vi "Ethernet Reader Modified.vi"() -> ()   [LabVIEW 2020]
doc: "This example creates a frame input stream session, reads frames at a set interval, and displays all the received frames from the latest read on the front panel."
uses:
  <resource>/objmgr/xnet.rc
  <vilib>/userdefined/xnetEnetEptRxFilterElement.ctl
  <vilib>/xnet/xnet.llb/XNET Create Session (Frame Input Stream).vi
  JLR/emea-tra-JLR-Synchronization-PoC/PoC_LV2020/States.ctl
  <vilib>/xnet/xnet.llb/XNET Read (State Time Current).vi
  JLR/emea-tra-JLR-Synchronization-PoC/PoC_LV2020/Data.ctl
  <vilib>/xnet/xnet.llb/XNET Read (Frame Ethernet).vi
  <vilib>/xnet/xnet.llb/XNET Read (State Time Trigger).vi
  <instrlib>/niSync/niSync.llb/niSync Set Time (Manual).vi
  <instrlib>/niSync/niSync.llb/niSync Initialize (Default).vi
  <vilib>/xnet/xnet.llb/XNET Frame Type Ethernet.ctl
  <vilib>/xnet/xnet.llb/XNET Frame Ethernet.ctl
panel:
  out "error out":errorcluster
  out "local time current":timestamp
  out "NI Sync Time":timestamp
  in  "Can Interface":refnum<k21>="LIN1"
  in  "Generate Trigger":bool
  out "Port State":u32(ring)=3 items=["Disabled"=3, "Master"=6, "Passive"=7, "Slave"=9]
  out "Synced?":bool
  out "Offset From Master (ns) 2":i64
  out "Frame Data (as hex string) Array 2":string[](array[string])
  out "Ethernet Read Frame Array 2":T1[](array[typedef]) {"fcs" format="%08x"; "network timestamp" format="%<%.7X\n%x>T"; "frame data" format="%x"; "local timestamp" format="%<%.7X\n%x>T"; "type" items=["Ethernet Data"=0, "Delay"=225, "Future Time Wait"=226]}
  out "Array Size 2":i32
  out "Number of Frames Received":u64
  in  "NI Sync Name":tag="Dev1"
  in  "Interface":refnum<k21>="ENET1"
  out "Time Diff (Sync vs Xnet) (s)":dbl format="%#.6f"
  in  "Stop 2":bool
  out "?":T3 {"Time Trigger Received" format="%<%.6X\n%x>T"}
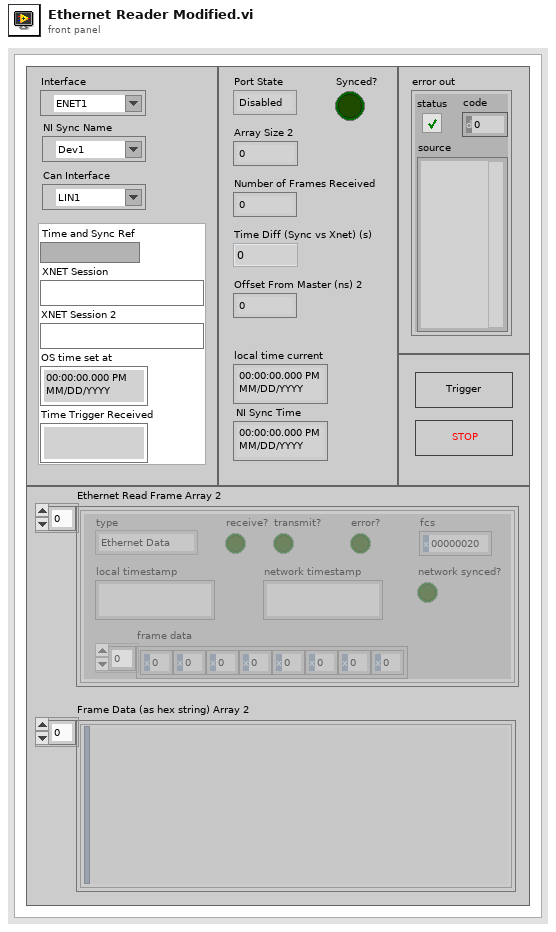
[diagram p1: front panel]
types:
  T1 = typedef "XNET Frame Ethernet.ctl" = cluster{"local timestamp":timestamp, "network timestamp":timestamp, "frame data":u8[], "fcs":u32, "type":T2, "network synced?":bool, "receive?":bool, "transmit?":bool, "error?":bool}
  T2 = typedef "XNET Frame Type Ethernet.ctl" = u16
  T3 = typedef "Data.ctl" = cluster{"Time and Sync Ref":refnum<k15>, "XNET Session":refnum<k21>, "XNET Session 2":refnum<k21>, "OS time set at":timestamp, "Time Trigger Received":timestamp}
  T4 = typedef "States.ctl" = enum16{"Init 8523", "Init 6683", "Sync 8523", "PPS+Trigger", "Set Sync Time", "Init 8510", "Adjust XNET time", "Idle", "Error"}
  T5 = typedef "xnetEnetEptRxFilterElement.ctl" = cluster{"use VID?":bool, "VID":u16, "use priority?":bool, "priority":u8, "use destination MAC?":bool, "destination MAC":string}
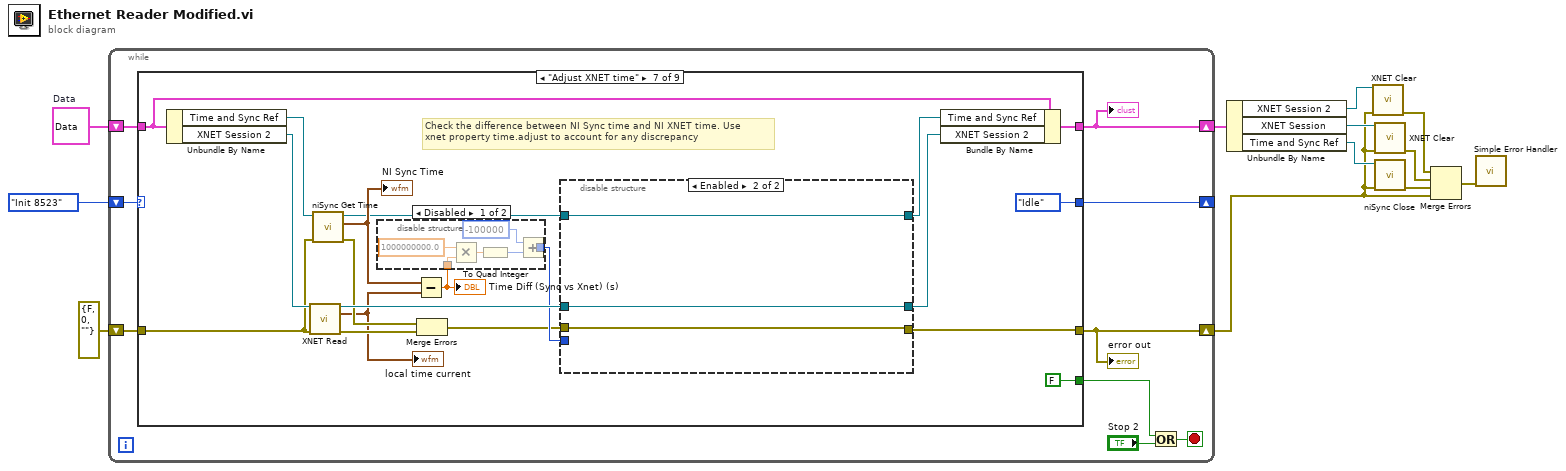
[diagram p0: block diagram]
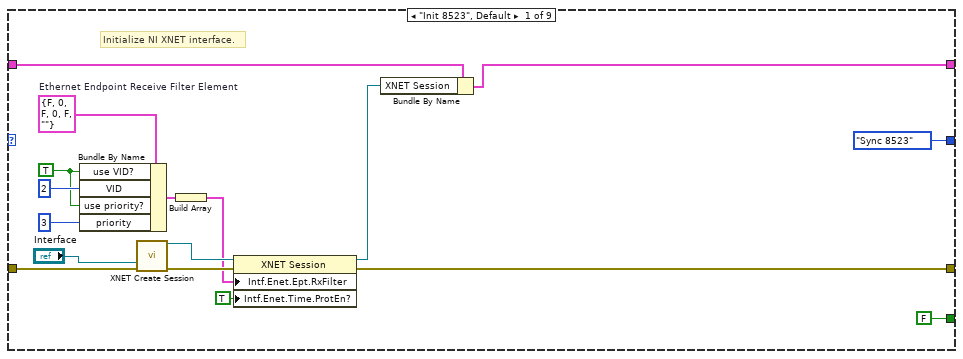
[diagram p2: hidden frame]
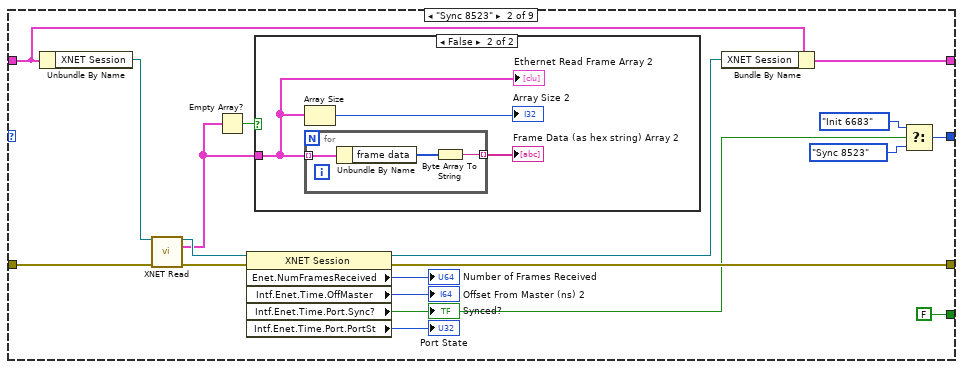
[diagram p3: hidden frame]
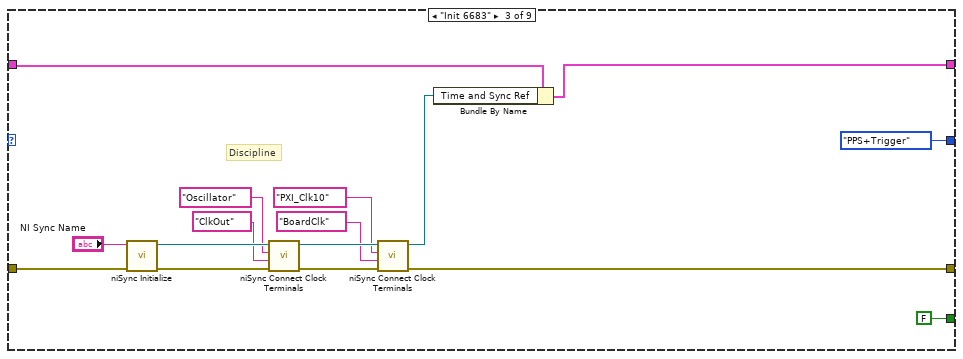
[diagram p5: hidden frame]
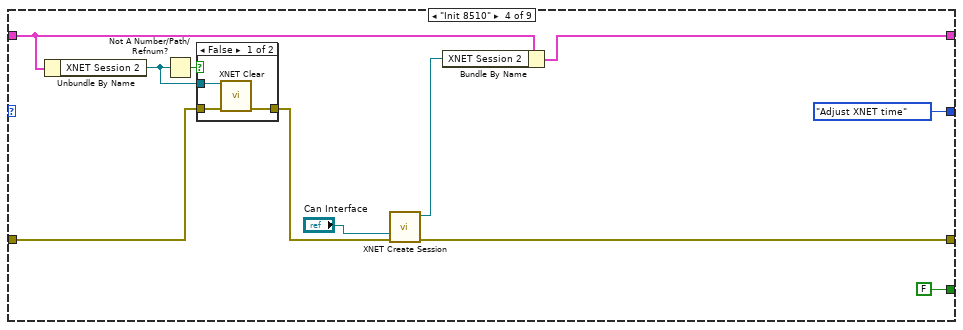
[diagram p6: hidden frame]
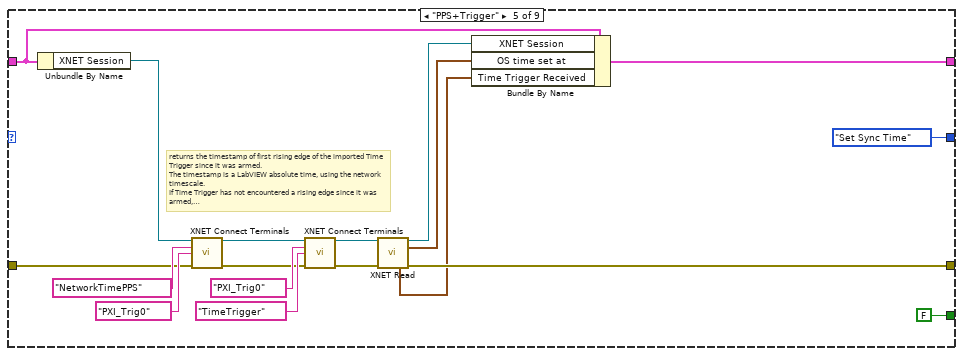
[diagram p8: hidden frame]
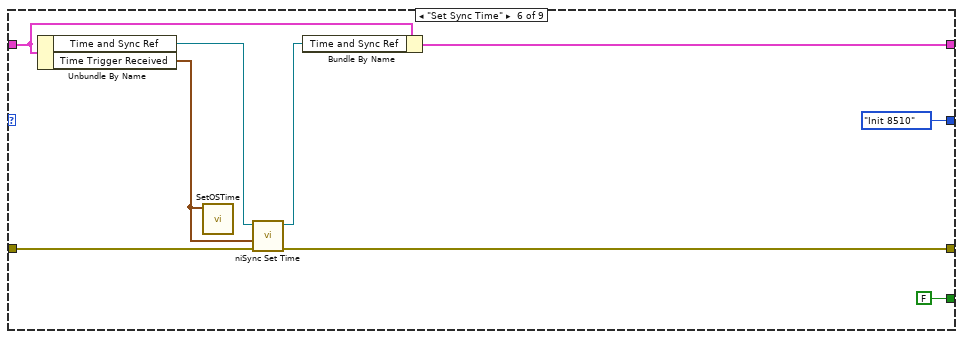
[diagram p9: hidden frame]
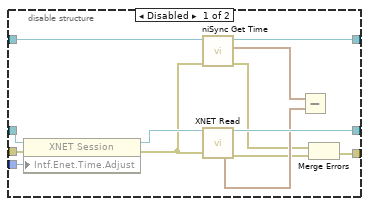
[diagram p11: hidden frame]
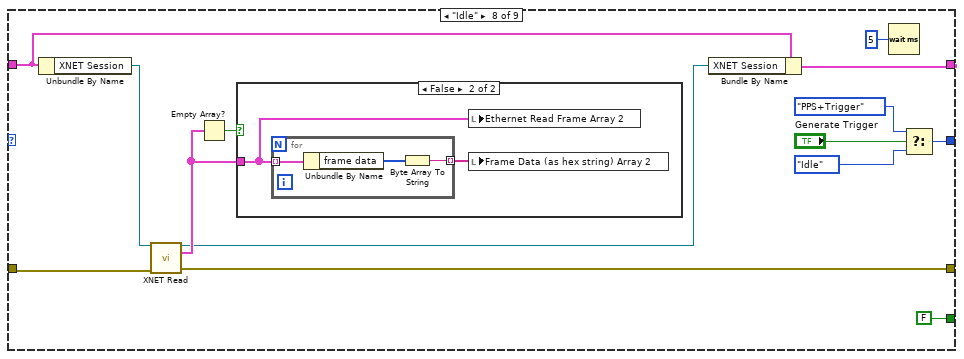
[diagram p12: hidden frame]
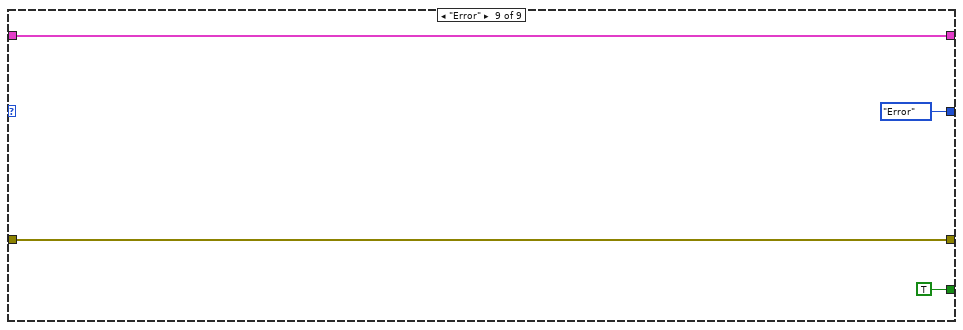
[diagram p14: hidden frame]
diagram:
  w6 = T3 {"Time and Sync Ref"="", "XNET Session"="", "XNET Session 2"="", "OS time set at"=timestamp(0 s since 1904-01-01), "Time Trigger Received"=timestamp(0 s since 1904-01-01)}  # Data
  n1 = while {
    shift-right: [w18] -> _
    shift-left: States."Init 8523" -> [w21]
    shift-right: [w13] -> w3
    shift-left: errorcluster {"status"=FALSE, "code"=0, "source"=""} ("error out") -> [w19]
    shift-right: [w15] -> w9
    shift-left: w6 -> [w20]
    stop <- w17 stop-if-true
    n2 = case shown="\"Adjust XNET time\"" w21 {
      tunnel: w20 -> [w38 w46 w69 w83 w101 w116 w124 w167 w181]
      tunnel: [w25 w52 w65 w86 w97 w115 w126 w165 w183] -> w13
      tunnel: w19 -> [w26 w43 w68 w80 w98 w118 w132 w166 w183]
      tunnel: [w36 w47 w67 w84 w100 w117 w133 w168 w181] -> w15
      tunnel: [States."Sync 8523" w49 States."PPS+Trigger" States."Adjust XNET time" States."Set Sync Time" States."Init 8510" States."Idle" w173 States."Error"] -> w18
      tunnel: [FALSE ("Intf.Enet.Time.Port.Sync?") FALSE ("Intf.Enet.Time.Port.Sync?") FALSE ("Intf.Enet.Time.Port.Sync?") FALSE ("Intf.Enet.Time.Port.Sync?") FALSE ("Intf.Enet.Time.Port.Sync?") FALSE ("Intf.Enet.Time.Port.Sync?") FALSE ("Intf.Enet.Time.Port.Sync?") FALSE ("Intf.Enet.Time.Port.Sync?") TRUE ("Intf.Enet.Time.Port.Sync?")] -> w14
      frame "Init 8523", Default {
        w28 = TRUE ("use VID?")
        w29 = T5 {"use VID?"=FALSE, "VID"=0, "use priority?"=FALSE, "priority"=0, "use destination MAC?"=FALSE, "destination MAC"=""}  # Ethernet Endpoint Receive Filter Element
        # "Initialize NI XNET interface."
        n3 = Bundle By Name(cluster=w29, "use VID?"=w28, "VID"=u16 2 ("VID 2"), "use priority?"=w28, "priority"=u8 3 ("priority 2")) -> (w32:T5)
        n4 = call-poly <vilib>:"XNET Create Session.vi"("interface"="Interface", "error in (no error)"=w26) -> ("session out"=w34:refnum<k21>, "error out"=w35:errorcluster)  [unwired: 12 in]
        n5 = Build Array(w32) -> (w33:T5[])
        n6 = property class="XNET Session"(reference=w34, error in=w35, "Intf.Enet.Ept.RxFilter"=w33, "Intf.Enet.Time.ProtEn?"=TRUE ("Interface:Ethernet:Time Sync:Protocol Enabled?")) -> (reference out=w24:refnum<k21>, error out=w25:errorcluster)
        n7 = Bundle By Name(cluster=w38, "XNET Session"=w24) -> (w36:T3)
      }
      frame "Sync 8523" {
        n8 = Unbundle By Name(w46) -> ("XNET Session"=w45:refnum<k21>)
        n9 = call-poly <vilib>:"XNET Read.vi"("session in"=w45, "error in (no error)"=w43) -> ("session out"=w42:refnum<k21>, "data"=w41:T1[], "error out"=w44:errorcluster)  [unwired: 10 in, 1 out]
        n10 = Empty Array?(array=w41) -> (empty?=w55:bool)
        n11 = property class="XNET Session"(reference=w42, error in=w44) -> (reference out=w48:refnum<k21>, error out=w52:errorcluster, "Enet.NumFramesReceived"=→"Number of Frames Received":u64, "Intf.Enet.Time.OffMaster"=→"Offset From Master (ns) 2":i64, "Intf.Enet.Time.Port.Sync?"=w40:bool, "Intf.Enet.Time.Port.PortSt"=→"Port State":u32)
        "Synced?" <- w40
        n12 = case shown="False" w55 {
          tunnel: w41 -> [_ w57]
          frame True {
          }
          frame False {
            n13 = Array Size(array=w57) -> (size(s)=→"Array Size 2":i32)
            n14 = for {
              tunnel: [w62] -> w59 mode=indexing
              tunnel: w57 -> [w61] mode=indexing
              n15 = Unbundle By Name(w61) -> ("frame data"=w60:u8[])
              n16 = Byte Array To String(unsigned byte array=w60) -> (string=w62:string)
            }
            "Frame Data (as hex string) Array 2" <- w59
            "Ethernet Read Frame Array 2" <- w57
          }
        }
        n17 = Bundle By Name(cluster=w46, "XNET Session"=w48) -> (w47:T3)
        n18 = Select(t=States."Init 6683", s=w40, f=States."Sync 8523") -> (s? t:f=w49:T4)
      }
      frame "Init 6683" {
        # "Discipline"
        n19 = call-poly <instrlib>:"niSync Initialize.vi"("error in (no error)"=w68, "resource name"="NI Sync Name") -> ("error out"=w78:errorcluster, "instrument handle out"=w77:refnum<k15>)  [unwired: 8 in]
        n20 = call <instrlib>:"niSync Connect Clock Terminals.vi"("error in (no error)"=w78, "destination terminal"="ClkOut", "source terminal"="Oscillator", "instrument handle"=w77) -> ("error out"=w75:errorcluster, "instrument handle out"=w76:refnum<k15>)  [unwired: 6 in]
        n21 = call <instrlib>:"niSync Connect Clock Terminals.vi"("error in (no error)"=w75, "destination terminal"="BoardClk", "source terminal"="PXI_Clk10", "instrument handle"=w76) -> ("error out"=w65:errorcluster, "instrument handle out"=w64:refnum<k15>)  [unwired: 6 in]
        n22 = Bundle By Name(cluster=w69, "Time and Sync Ref"=w64) -> (w67:T3)
      }
      frame "Init 8510" {
        n23 = Unbundle By Name(w83) -> ("XNET Session 2"=w81:refnum<k21>)
        n24 = Not A Number/Path/Refnum?(number/path/refnum=w81) -> (NaN/Path/Refnum?=w82:bool)
        n25 = case shown="False" w82 {
          tunnel: w81 -> [w92 _]
          tunnel: w80 -> [w91 w93]
          tunnel: [w90 w93] -> w79
          frame False {
            n26 = call <vilib>:"XNET Clear.vi"("session in"=w92, "error in (no error)"=w91) -> ("error out"=w90:errorcluster)  [unwired: 13 in]
          }
          frame True {
          }
        }
        n27 = call-poly <vilib>:"XNET Create Session.vi"("interface"="Can Interface", "error in (no error)"=w79) -> ("session out"=w85:refnum<k21>, "error out"=w86:errorcluster)  [unwired: 1 in, 11 out]
        n28 = Bundle By Name(cluster=w83, "XNET Session 2"=w85) -> (w84:T3)
      }
      frame "PPS+Trigger" {
        # "returns the timestamp of first rising edge of the imported Time Trigger since it was armed. \nThe timestamp is a LabVIEW absolute time, using the network timescale. \nIf Time Trigger has not encountered a rising edge since it was armed, \nnetwork time trigger returns zero (an invalid timestamp)."
        n29 = Unbundle By Name(w101) -> ("XNET Session"=w103:refnum<k21>)
        n30 = call <vilib>:"XNET Connect Terminals.vi"("session in"=w103, "source terminal"=tag "NetworkTimePPS", "destination terminal"=tag "PXI_Trig0", "error in (no error)"=w98) -> ("session out"=w106:refnum<k21>, "error out"=w107:errorcluster)  [unwired: 10 in]
        n31 = call <vilib>:"XNET Connect Terminals.vi"("session in"=w106, "source terminal"=tag "PXI_Trig0", "destination terminal"=tag "TimeTrigger", "error in (no error)"=w107) -> ("session out"=w102:refnum<k21>, "error out"=w104:errorcluster)  [unwired: 10 in]
        n32 = call-poly <vilib>:"XNET Read.vi"("session in"=w102, "error in (no error)"=w104) -> ("session out"=w111:refnum<k21>, "local time trigger"=w95:timestamp, "network time trigger"=w94:timestamp, "error out"=w97:errorcluster)  [unwired: 9 in, 1 out]
        n33 = Bundle By Name(cluster=w101, "XNET Session"=w111, "OS time set at"=w95, "Time Trigger Received"=w94) -> (w100:T3)
      }
      frame "Set Sync Time" {
        n34 = Unbundle By Name(w116) -> ("Time and Sync Ref"=w119:refnum<k15>, "Time Trigger Received"=w112:timestamp)
        n35 = call "SetOSTime.vi"("OS time"=w112) -> ()  [unwired: 10 in, 1 out]
        n36 = call-poly <instrlib>:"niSync Set Time.vi"("error in (no error)"=w118, "initial time"=w112, "instrument handle"=w119) -> ("error out"=w115:errorcluster, "instrument handle out"=w114:refnum<k15>)  [unwired: 7 in]
        n37 = Bundle By Name(cluster=w116, "Time and Sync Ref"=w114) -> (w117:T3)
      }
      frame "Adjust XNET time" {
        # "Check the difference between NI Sync time and NI XNET time. Use\nxnet property time.adjust to account for any discrepancy"
        n38 = Unbundle By Name(w124) -> ("Time and Sync Ref"=w134:refnum<k15>, "XNET Session 2"=w135:refnum<k21>)
        n39 = call-poly <vilib>:"XNET Read.vi"("session in"=w135, "error in (no error)"=w132) -> ("session out"=w137:refnum<k21>, "local time current"=w123:timestamp, "error out"=w136:errorcluster)  [unwired: 9 in, 2 out]
        "local time current" <- w123
        n40 = call <instrlib>:"niSync Get Time.vi"("error in (no error)"=w132, "instrument handle"=w134) -> ("error out"=w131:errorcluster, "time"=w139:timestamp, "instrument handle out"=w128:refnum<k15>)  [unwired: 5 in]
        "NI Sync Time" <- w139
        n41 = Subtract(x=w139, y=w123) -> (x-y=w138:dbl)
        "Time Diff (Sync vs Xnet) (s)" <- w138
        n42 = disable-structure shown="Disabled" {
          disable-tunnel: w138 -> [w145 _]
          disable-tunnel: [w141 _] -> w125
          frame Disabled {
            n43 = Multiply(x=1000000000.0 ("y"), y=w145) -> (x*y=w143:dbl)
            n44 = To Quad Integer(1:w143) -> (0:w142:i64)
            n45 = Add(x=i64 -100000, y=w142) -> (x+y=w141:i64)
          }
          frame Enabled {
          }
        }
        n46 = Merge Errors(w131, w136) -> (w121:errorcluster)
        n47 = disable-structure shown="Enabled" {
          disable-tunnel: w137 -> [w158 w160]
          disable-tunnel: [w156 w160] -> w129
          disable-tunnel: w128 -> [w155 w161]
          disable-tunnel: [w153 w161] -> w127
          disable-tunnel: [w149 w159] -> w126
          disable-tunnel: w125 -> [w148 _]
          disable-tunnel: w121 -> [w147 w159]
          frame Disabled {
            n48 = property class="XNET Session"(reference=w158, error in=w147, "Intf.Enet.Time.Adjust"=w148) -> (reference out=w157:refnum<k21>, error out=w146:errorcluster)
            n49 = call <instrlib>:"niSync Get Time.vi"("error in (no error)"=w146, "instrument handle"=w155) -> ("error out"=w150:errorcluster, "time"=w154:timestamp, "instrument handle out"=w153:refnum<k15>)  [unwired: 5 in]
            n50 = call-poly <vilib>:"XNET Read.vi"("session in"=w157, "error in (no error)"=w146) -> ("session out"=w156:refnum<k21>, "network time current"=w152:timestamp, "error out"=w151:errorcluster)  [unwired: 9 in, 2 out]
            n51 = Subtract(x=w154, y=w152) -> ()  [unwired: 1 out]
            n52 = Merge Errors(w150, w151) -> (w149:errorcluster)
          }
          frame Enabled {
          }
        }
        n53 = Bundle By Name(cluster=w124, "Time and Sync Ref"=w127, "XNET Session 2"=w129) -> (w133:T3)
      }
      frame "Idle" {
        n54 = Unbundle By Name(w167) -> ("XNET Session"=w170:refnum<k21>)
        n55 = call-poly <vilib>:"XNET Read.vi"("session in"=w170, "error in (no error)"=w166) -> ("session out"=w164:refnum<k21>, "data"=w169:T1[], "error out"=w165:errorcluster)  [unwired: 10 in, 1 out]
        n56 = Empty Array?(array=w169) -> (empty?=w171:bool)
        n57 = case shown="False" w171 {
          tunnel: w169 -> [_ w177]
          frame True {
          }
          frame False {
            n58 = for {
              tunnel: [w180] -> w176 mode=indexing
              tunnel: w177 -> [w179] mode=indexing
              n59 = Unbundle By Name(w179) -> ("frame data"=w178:u8[])
              n60 = Byte Array To String(unsigned byte array=w178) -> (string=w180:string)
            }
            n61 = local write "Ethernet Read Frame Array 2"(w177) -> ()
            n62 = local write "Frame Data (as hex string) Array 2"(w176) -> ()
          }
        }
        n63 = Bundle By Name(cluster=w167, "XNET Session"=w164) -> (w168:T3)
        n64 = Wait (ms)(milliseconds to wait=u32 5) -> ()  [unwired: 1 out]
        n65 = Select(t=States."PPS+Trigger", s="Generate Trigger", f=States."Idle") -> (s? t:f=w173:T4)
      }
      frame "Error" {
      }
    }
    "?" <- w15
    "error out" <- w13
    n66 = Or(x=w14, y="Stop 2") -> (x .or. y?=w17:bool)
  }
  n67 = Unbundle By Name(w9) -> ("XNET Session 2"=w4:refnum<k21>, "XNET Session"=w8:refnum<k21>, "Time and Sync Ref"=w7:refnum<k15>)
  n68 = call <vilib>:"XNET Clear.vi"("session in"=w4, "error in (no error)"=w3) -> ("error out"=w2:errorcluster)  [unwired: 13 in]
  n69 = call <vilib>:"XNET Clear.vi"("session in"=w8, "error in (no error)"=w3) -> ("error out"=w12:errorcluster)  [unwired: 13 in]
  n70 = call <instrlib>:"niSync Close.vi"("error in (no error)"=w3, "instrument handle"=w7) -> ("error out"=w10:errorcluster)  [unwired: 9 in]
  n71 = Merge Errors(w2, w12, w10, w3) -> (w11:errorcluster)
  n72 = call <vilib>:"Simple Error Handler.vi"("error in (no error)"=w11) -> ()  [unwired: 4 in, 5 out]
